vi "DoDrawSprites.vi"(8 "error in (no error)":errorcluster, 10 "Sprites in":T1, 11 "Game in":refnum<class "Game.lvclass">) -> (0 "error out":errorcluster, 2 "Sprites out":T1, 3 "Game out":refnum<class "Game.lvclass">)   [LabVIEW 2019, in "RT_Game.lvlib" / "Game.lvclass"]
uses:
  Game.lvclass
  SpritesCluster.ctl
  RT_Sprite/RT_Sprite.lvclass
  Game.lvclass/Game.ctl
  RT_Sprite/RT_Sprite.lvclass/RT_Sprite.ctl
  RT_Sprite/Read Picture.vi
  Read FPGA_ref.vi
  Write FPGA_ref.vi
  <vilib>/Utility/error.llb/Error Cluster From Error Code.vi
  <vilib>/rvi/errors/niLvFpgaAdjustHostInterfaceError.vi
  FPGA_Interface.ctl
  <vilib>/rvi/interface/nirviReadWriteControl/nirviReadWriteControl.xnode
  FPGA Bitfiles/myriogameconsole_FPGATarget_Main_ntsPRcBZGxk.lvbitx
  <vilib>/rvi/interface/nirviMethod/nirviMethod.xnode
  NiFpgaLv.dll
  <vilib>/FPGAPlugInAG/myRIO-1900/niLvFpga_WriteFifo_myRIO-1900.vi
  <vilib>/rvi/errors/niLvFpgaMergeErrorWithErrorCode.vi
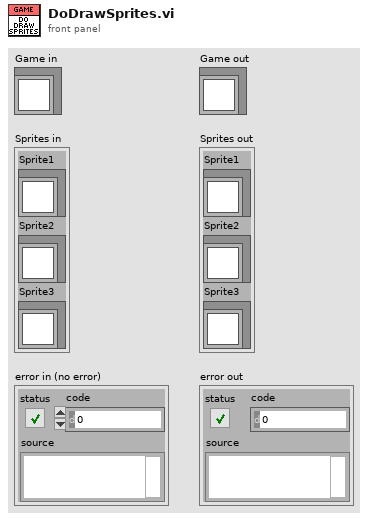
[diagram p1: front panel]
types:
  T1 = typedef "RT_Game.lvlib/Game.lvclass/SpritesCluster.ctl" = cluster{"Sprite1":refnum<class "RT_Sprite.lvclass">, "Sprite2":refnum<class "RT_Sprite.lvclass">, "Sprite3":refnum<class "RT_Sprite.lvclass">}
  T2 = typedef "FPGA_Interface.ctl" = refnum<k20>
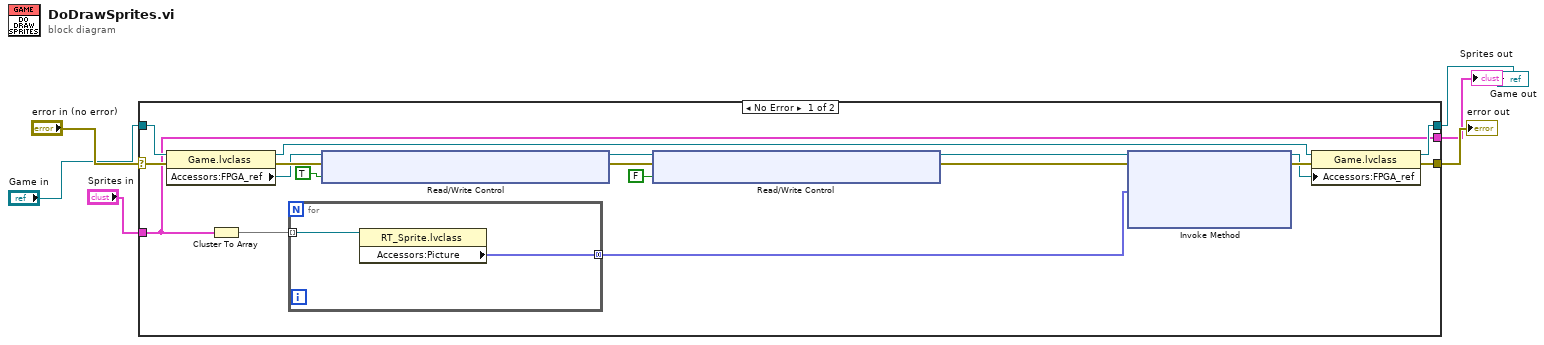
[diagram p0: block diagram]
diagram:
  n1 = case shown="No Error" "error in (no error)" {
    selector: "error in (no error)" -> [w20 w29]
    tunnel: [w21 w29] -> w5
    tunnel: [w10 w28] -> w2
    tunnel: "Sprites in" -> [w10 w28]
    tunnel: [w23 w27] -> w1
    tunnel: "Game in" -> [w24 w27]
    frame No Error {
      n2 = property class="Game.lvclass"(reference=w24, error in=w20) -> (reference out=w9:refnum<class "Game.lvclass">, error out=w22:errorcluster, "Accessors:FPGA_ref"=w15:T2)
      n3 = Cluster To Array(cluster=w10) -> (array=w7:refnum<class "RT_Sprite.lvclass">[])
      n4 = for {
        tunnel: w7 -> [w26] mode=indexing
        tunnel: [w25] -> w17 mode=concatenating
        n5 = property class="RT_Sprite.lvclass"(reference=w26) -> ("Accessors:Picture"=w25:fxp<+,3,3>[])  [unwired: 1 in, 2 out]
      }
      n6 = xnode "Read/Write Control"("FPGA VI Reference In"=w15, "error in"=w22, "Spritebuffer_ResetAddress"=TRUE) -> ("FPGA VI Reference Out"=w12:T2, "error out"=w16:errorcluster)
      n7 = xnode "Read/Write Control"("FPGA VI Reference In"=w12, "error in"=w16, "Spritebuffer_ResetAddress"=FALSE) -> ("FPGA VI Reference Out"=w11:T2, "error out"=w14:errorcluster)
      n8 = xnode "Invoke Method"("FPGA VI Reference In"=w11, "error in"=w14, "Data"=w17) -> ("FPGA VI Reference Out"=w18:T2, "error out"=w19:errorcluster)  [unwired: 1 in, 1 out]
      n9 = property class="Game.lvclass"(reference=w9, error in=w19, "Accessors:FPGA_ref"=w18) -> (reference out=w23:refnum<class "Game.lvclass">, error out=w21:errorcluster)
    }
    frame Error {
    }
  }
  "error out" <- w5
  "Sprites out" <- w2
  "Game out" <- w1
